vi "svx_Orbit Notation.vi"(4 "probe angles":cluster{"angles X":dbl, "angles Y":dbl}, 10 "Plot Area:Size":T1={"Width"=100, "Height"=100}, 11 "Picture in":picture) -> (1 "text max size":i16, 2 "Plot Area:Size out":T1={"Width"=100, "Height"=100}, 3 "Picture out":picture)   [LabVIEW 2017, in "SVX Orbit.xctl"]
uses:
  <vilib>/addons/_XControls/Orbit Plot/SVX Orbit.xctl
  <vilib>/Utility/miscctls.llb/LVBoundsTypeDef.ctl
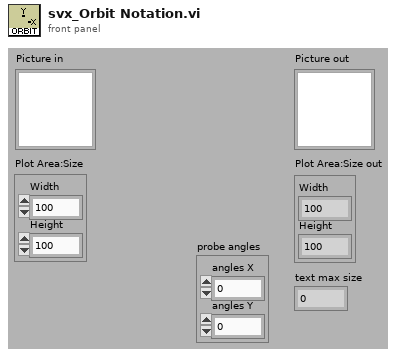
[diagram p1: front panel]
types:
  T1 = typedef "LVBoundsTypeDef.ctl" = cluster{"Width":u32, "Height":u32}
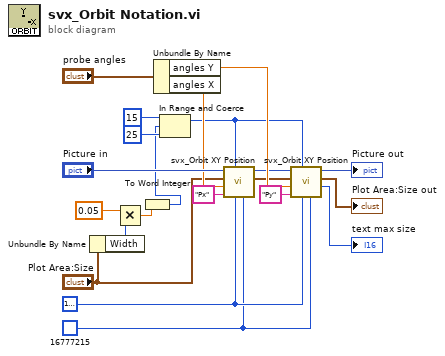
[diagram p0: block diagram]
diagram:
  w11 = u32 16777222 ("Text Color")
  w10 = u32 16777215 ("Text Color")
  n1 = Unbundle By Name("Plot Area:Size") -> ("Width"=w6:u32)
  n2 = Multiply(x=0.05, y=w6) -> (x*y=w2:dbl)
  n3 = To Word Integer(number=w2) -> (16bit integer=w1:i16)
  n4 = Unbundle By Name("probe angles") -> ("angles Y"=w17:dbl, "angles X"=w19:dbl)
  n5 = In Range and Coerce(upper limit=i16 15 ("Size"), x=w1, lower limit=i16 25) -> (coerced(x)=w4:i16)  [unwired: 1 out]
  n6 = call <vilib>:"svx_Orbit XY Position.vi"("text color"=w10, "BG color"=w11, "Size"=w4, "text"="Px", "angle (rad)"=w19, "Plot Area:Size"="Plot Area:Size", "Picture in"="Picture in") -> ("Plot Area:Size out"=w15:T1, "Picture out"=w16:picture)  [unwired: 2 in, 1 out]
  n7 = call <vilib>:"svx_Orbit XY Position.vi"("text color"=w10, "BG color"=w11, "Size"=w4, "text"="Py", "angle (rad)"=w17, "Plot Area:Size"=w15, "Picture in"=w16) -> ("text max size"=→"text max size":i16, "Plot Area:Size out"=→"Plot Area:Size out":T1, "Picture out"=→"Picture out":picture)  [unwired: 2 in]
